vi "ziExample-HF2-Noise.vi"() -> ()   [LabVIEW 2009]
doc: "Control a Zurich instrument device via the LabOne Labview API. \nRequirements: Zurich Instruments HF2.\n\nThis is an example for a Zurich Instruments HF2 instrument. This example VI calculates the rms noise and the noise spectral densitiy of the input signal at a certain demodulator frequency. \n\nThe VI performs the following steps:\n(1) Load the settings file or, adjust the required settings in ziControl. Set the required demodulator frequency and the required time constant / bandwidth. \n(2) the VI subrscribes to the corresponding demodulator (this demodulator needs to be switched on in the user manual, otherwise no data is received) \n(3) the data is acquired/polled and the RMS noise is calculated by using the following equation:\n RMSnoise = RMS(X - Xmean), RMS stands for root-mean-square\n the number of averages can be chosen by the user \n\n© Zurich Instruments AG, www.zhinst.com"
uses:
  <vilib>/measure/madcrms.llb/Basic Averaged DC-RMS for 1 Chan.vi
  <instrlib>/Zurich Instruments LabOne/Zurich Instruments LabOne.lvlib
  <vilib>/measure/NI_MAPro.lvlib
panel:
  out "Error Out":errorcluster
  out "Sel. Device":string
  in  "Address":string="DEV"
  in  "Averaging":i32=100 min=0 max=1024 step=1
  in  "ReadSettingsFile":bool=TRUE caption="Read Settings File"
  out "BW":dbl=9.729925316888316 format="%#_6p"
  out "Ref Freq [Hz]":dbl=1141592.6499998362 format="%#_6p"
  out "Noise Spectral Density\nVrms/sqrt(Hz)":dbl=1.331104953906021e-08 format="%0.2p"
  in  "X or Y":u16(ring) items=["Xnoise", "Ynoise", "Rnoise"]
  out "RMS Value":dbl(graph)=4.1520928155609186e-08
  out "RMS noise":dbl=4.1520928155609186e-08 format="%0.2p"
  in  "Demodulator":u16(ring) items=["Demod 1", "Demod 2", "Demod 3", "Demod 4", "Demod 5", "Demod 6"]
  in  "stop":bool
  # "HF2 Example Noise Measurement.vi\nRequirements: HF2, ziControl for settings, \nZurich Instruments LabVIEW API. \nsee block diagram for VI description"
  # "Tested Devices:\n- HF2LI\nIncompatible Device:\n- UHFLI (wrong BW calcualtions)"
  # "Settings"
  # "Output"
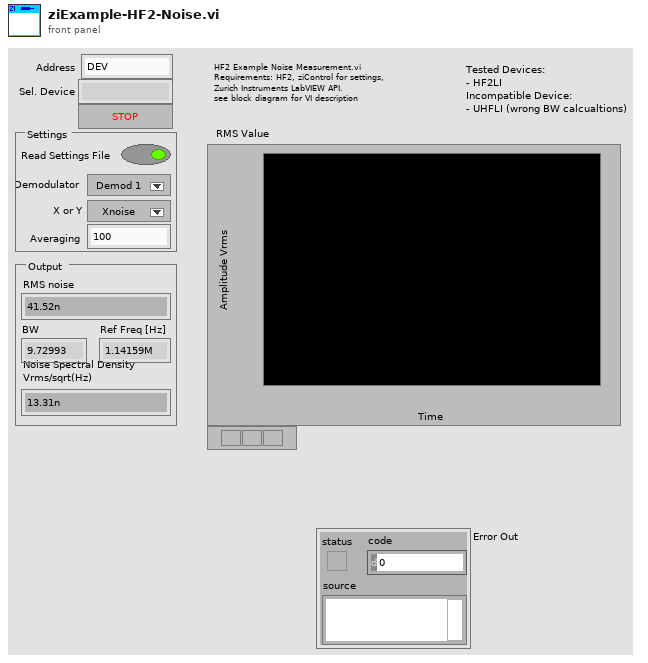
[diagram p1: front panel]
types:
  T1 = typedef "Zurich Instruments LabOne.lvlib/ziTypeHandle.ctl" = cluster{"handleValid":bool, "Conn":u64, "Path Prefix":string, "Handle":u64, "Connected":bool, "Clockbase(s)":dbl}
  T2 = typedef "Zurich Instruments LabOne.lvlib/ziTypePollData.ctl" = cluster{"double":dbl, "Demod Sample":T3, "string":string, "Raw":u8[], "int":i32, "ScopeData":cluster{"wave":i16[], "dt (s)":dbl}, "DioInput":cluster{"Timestamp (ticks)":u64[], "Value":u32[]}, "AuxInput":cluster{"Timestamp (ticks)":u64[], "Val Ch0 (V)":dbl[], "Val Ch1 (V)":dbl[]}}
  T3 = typedef "Zurich Instruments LabOne.lvlib/ziTypeDemodSample.ctl" = cluster{"Channel":i32, "Timestamps (ticks)":u64[], "X (Vrms)":dbl[], "Y (Vrms)":dbl[], "Osc Phase (deg)":dbl[], "Freq (Hz)":dbl[], "DIO":u32[], "Aux In 0 (V)":dbl[], "Aux In 1 (V)":dbl[]}
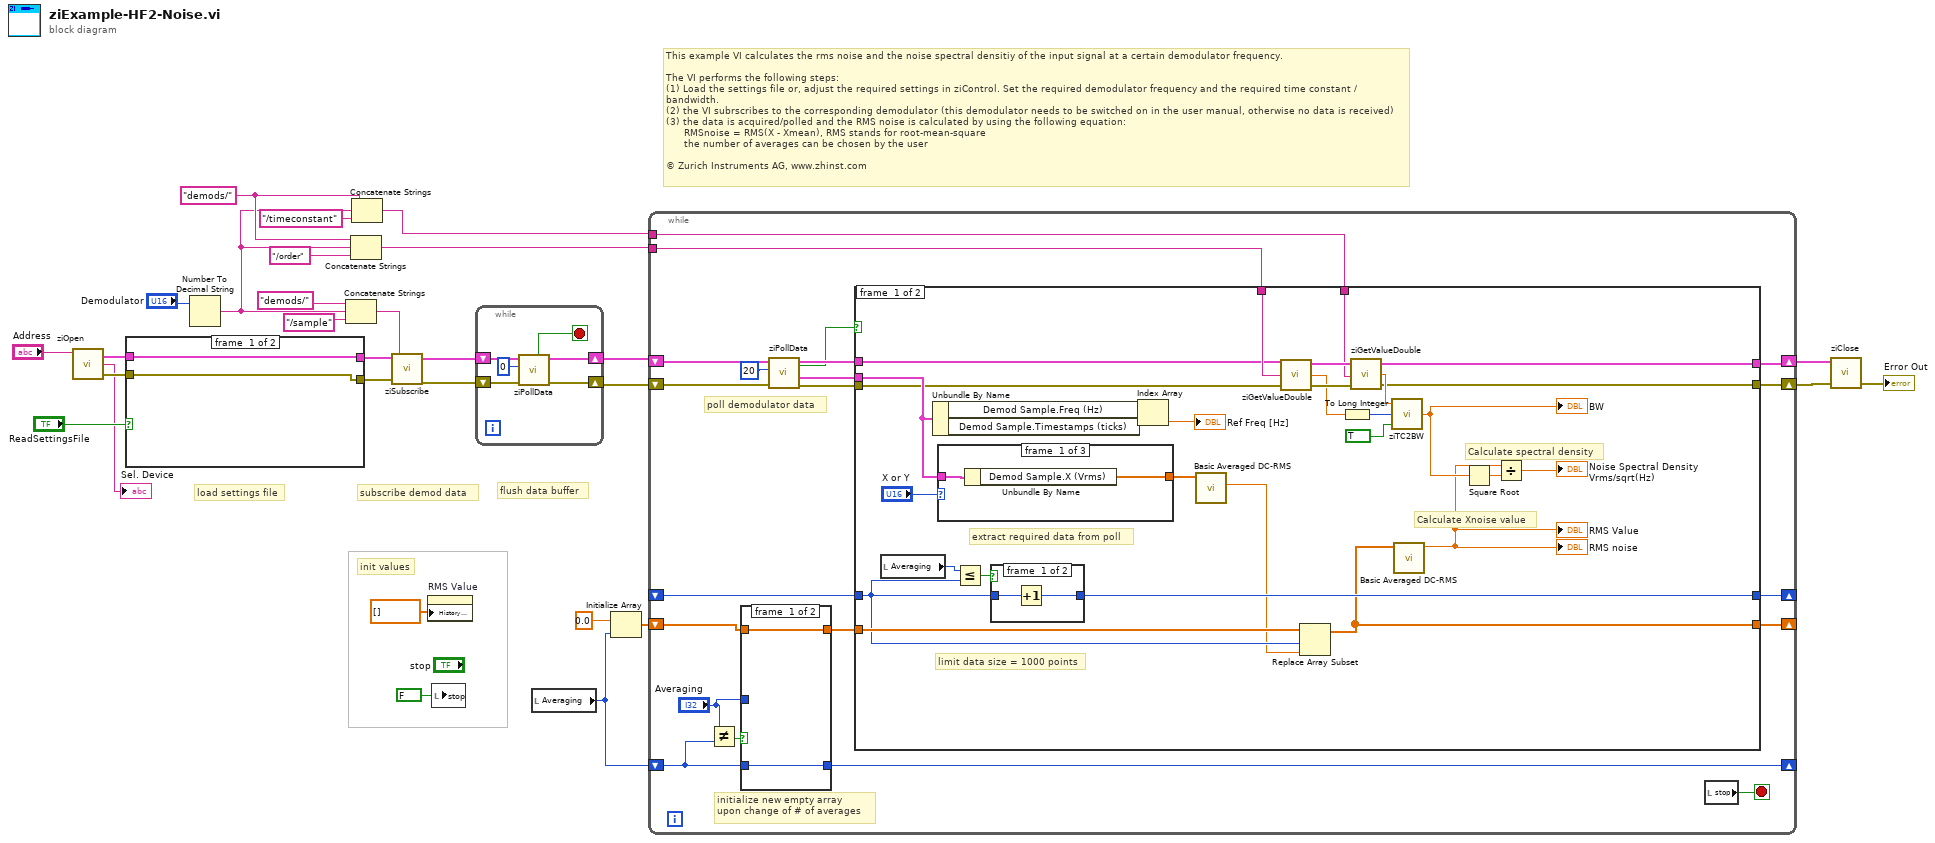
[diagram p0: block diagram]
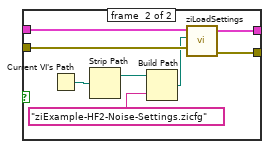
[diagram p2: hidden frame]
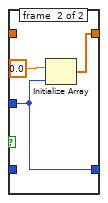
[diagram p3: hidden frame]
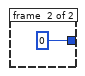
[diagram p4: hidden frame]
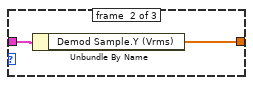
[diagram p5: hidden frame]
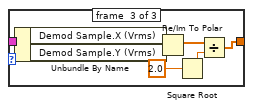
[diagram p6: hidden frame]
diagram:
  w18 = "demods/" ("path")
  # "load settings file"
  # "flush data buffer"
  # "init values"
  # "subscribe demod data"
  # "This example VI calculates the rms noise and the noise spectral densitiy of the input signal at a certain demodulator frequency. \n\nThe VI performs the following steps:\n(1) Load the settings file or, adjust the required settings in ziControl. Set the required demodulator frequency and the required time constant / bandwidth. \n(2) the VI subrscribes to the corresponding demodulator (this demodulator needs to be switched on in the user manual, otherwise no data is received)  \n(3) the data is acquired/polled and the RMS noise is calculated by using the following equation:\n      RMSnoise = RMS(X - Xmean), RMS stands for root-mean-square\n      the number of averages can be chosen by the user \n\n© Zurich Instruments AG, www.zhinst.com"
  n1 = call <instrlib>:"ziOpen.vi"("Address"="Address") -> ("Error Out"=w11:errorcluster, "Selected Device"=→"Sel. Device":string, "HandleOut"=w12:T1)  [unwired: 1 in, 2 out]
  n2 = case shown="True" "ReadSettingsFile" {
    tunnel: w12 -> [w31 w39]
    tunnel: w11 -> [w30 w38]
    tunnel: [w31 w37] -> w10
    tunnel: [w30 w36] -> w9
    frame #0 {
    }
    frame #1 {
      n3 = Current VI's Path() -> (path=w32:path)
      n4 = Strip Path(path=w32) -> (stripped path=w33:path)  [unwired: 1 out]
      n5 = Build Path(base path=w33, name or relative path="ziExample-HF2-Noise-Settings.zicfg" ("path")) -> (appended path=w34:path)
      n6 = call <instrlib>:"ziLoadSettings.vi"("Error in"=w38, "File path (dialog if empty)"=w34, "Handle in"=w39) -> ("Error out"=w36:errorcluster, "Handle out"=w37:T1)  [unwired: 2 in]
    }
  }
  n7 = Number To Decimal String(number="Demodulator") -> (decimal integer string=w7:string)  [unwired: 1 out]
  n8 = Concatenate Strings("demods/" ("path"), w7, "/sample" ("path")) -> (w25:string)
  n9 = Concatenate Strings(w18, w7, "/order" ("path")) -> (w23:string)
  n10 = Concatenate Strings(w18, w7, "/timeconstant" ("path")) -> (w22:string)
  n11 = call <instrlib>:"ziSubscribe.vi"("error in"=w9, "Path ()"=w25, "Handle In"=w10) -> ("error out"=w15:errorcluster, "Handle Out"=w16:T1)  [unwired: 1 in]
  n12 = property on="RMS Value" class="WFChart (strict)"("History Data"=dbl[] []) -> ()  [unwired: 2 in, 2 out]
  n13 = local write "stop"(FALSE ("Record")) -> ()
  n14 = while {
    shift-right: [w43] -> w14
    shift-left: w16 -> [w45]
    shift-right: [w42] -> w13
    shift-left: w15 -> [w44]
    stop <- w40 stop-if-true
    n15 = call <instrlib>:"ziPollData.vi"("Error In"=w44, "TimeOut ms (50)"=0, "Handle In"=w45) -> ("Error Out"=w42:errorcluster, "Handle Out"=w43:T1, "Timed Out"=w40:bool)  [unwired: 1 in, 5 out]
  }
  n16 = local read "Averaging"() -> (w4:i32)
  n17 = Initialize Array(0.0 ("element"), w4) -> (w6:dbl[])
  n18 = while {
    shift-right: [w59] -> w29
    shift-left: w14 -> [w66]
    shift-right: [w58] -> w28
    shift-left: w13 -> [w65]
    shift-right: [w52] -> _
    shift-left: w6 -> [w51]
    tunnel: w23 -> [w56]
    tunnel: w22 -> [w57]
    shift-right: [w53] -> _
    shift-left: _ -> [w54]
    shift-right: [w47] -> _
    shift-left: w4 -> [w46]
    stop <- w63 stop-if-true
    # "initialize new empty array\nupon change of # of averages"
    # "poll demodulator data"
    n19 = Not Equal?(x="Averaging", y=w46) -> (x != y?=w49:bool)
    n20 = case shown="False" w49 {
      tunnel: w51 -> [w68 _]
      tunnel: [w68 w70] -> w50
      tunnel: "Averaging" -> [_ w69]
      tunnel: [w67 w69] -> w47
      tunnel: w46 -> [w67 _]
      frame #0 {
      }
      frame #1 {
        n21 = Initialize Array(0.0 ("element"), w69) -> (w70:dbl[])
      }
    }
    n22 = call <instrlib>:"ziPollData.vi"("Error In"=w65, "TimeOut ms (50)"=20, "Handle In"=w66) -> ("Error Out"=w60:errorcluster, "Data Out"=w62:T2, "Handle Out"=w61:T1, "Timed Out"=w55:bool)  [unwired: 1 in, 4 out]
    n23 = case shown="False" w55 {
      tunnel: w62 -> [w96 _]
      tunnel: w61 -> [w76 w117]
      tunnel: w60 -> [w75 w116]
      tunnel: [w86 w117] -> w59
      tunnel: [w85 w116] -> w58
      tunnel: w57 -> [w93 _]
      tunnel: w56 -> [w88 _]
      tunnel: [w80 w114] -> w52
      tunnel: w54 -> [w78 w115]
      tunnel: [w84 w115] -> w53
      tunnel: w50 -> [w79 w114]
      frame #0 {
        # "extract required data from poll"
        # "Calculate spectral density"
        # "Calculate Xnoise value"
        # "limit data size = 1000 points"
        n24 = local read "Averaging"() -> (w81:i32)
        n25 = Unbundle By Name(w96) -> ("Demod Sample.Freq (Hz)"=w87:dbl[])  [unwired: 1 out]
        n26 = case shown="2" "X or Y" {
          tunnel: w96 -> [w104 w105 w113]
          tunnel: [w103 w106 w109] -> w82
          frame #0 {
            n27 = Unbundle By Name(w104) -> ("Demod Sample.X (Vrms)"=w103:dbl[])
          }
          frame #1 {
            n28 = Unbundle By Name(w105) -> ("Demod Sample.Y (Vrms)"=w106:dbl[])
          }
          frame #2 {
            n29 = Unbundle By Name(w113) -> ("Demod Sample.X (Vrms)"=w112:dbl[], "Demod Sample.Y (Vrms)"=w111:dbl[])
            n30 = Re/Im To Polar(2:w111, 3:w112) -> (1:w110:dbl[])  [unwired: 1 out]
            n31 = Square Root(x=2.0) -> (sqrt(x)=w108:dbl)
            n32 = Divide(x=w110, y=w108) -> (x/y=w109:dbl[])
          }
        }
        n33 = Less Or Equal?(x=w81, y=w78) -> (x <= y?=w83:bool)
        n34 = case shown="True" w83 {
          tunnel: [w101 u32 0] -> w84
          tunnel: w78 -> [w100 _]
          frame #0 {
            n35 = Increment(x=w100) -> (x+1=w101:u32)
          }
          frame #1 {
          }
        }
        n36 = Index Array(array=w87) -> (element=→"Ref Freq [Hz]":dbl)  [unwired: 1 in]
        n37 = call-poly <vilib>:"Basic Averaged DC-RMS.vi"("signal in"=w82) -> ("RMS value"=w77:dbl)  [unwired: 4 in, 6 out]
        n38 = call <instrlib>:"ziGetValueDouble.vi"("error in"=w75, "Path"=w88, "Handle in"=w76) -> ("error out"=w95:errorcluster, "Value"=w90:dbl, "Handle out"=w94:T1)
        n39 = Replace Array Subset(array=w79, new element=w77, index=w78) -> (w80:dbl[])
        n40 = To Long Integer(number=w90) -> (32bit integer=w92:i32)
        n41 = call <instrlib>:"ziGetValueDouble.vi"("error in"=w95, "Path"=w93, "Handle in"=w94) -> ("error out"=w85:errorcluster, "Value"=w91:dbl, "Handle out"=w86:T1)
        n42 = call <instrlib>:"ziTC2BW.vi"("Eq BW (F)"=TRUE ("Eq BW"), "Order (1)"=w92, "TC (s)"=w91) -> ("BW (Hz)"=w89:dbl)
        "BW" <- w89
        n43 = call-poly <vilib>:"Basic Averaged DC-RMS.vi"("signal in"=w80) -> ("DC value"=w72:dbl)  [unwired: 4 in, 6 out]
        "RMS noise" <- w72
        "RMS Value" <- w72
        n44 = Square Root(x=w89) -> (sqrt(x)=w97:dbl)
        n45 = Divide(x=w72, y=w97) -> (x/y=→"Noise Spectral Density\nVrms/sqrt(Hz)":dbl)
      }
      frame #1 {
      }
    }
    n46 = local read "stop"() -> (w63:bool)
  }
  n47 = call <instrlib>:"ziClose.vi"("Error In"=w28, "Handle In"=w29) -> ("Error Out"=→"Error Out":errorcluster)  [unwired: 3 out]
